vi "Clean Shutdown Check (SubVI).vi"(7 "System Message Queue In":refnum<queue>, 8 "error in (no error)":errorcluster) -> (0 "error out":errorcluster)   [LabVIEW 2019]
uses:
  Globals and Definitions/System Message.ctl
  Globals and Definitions/Initialization Globals.vi
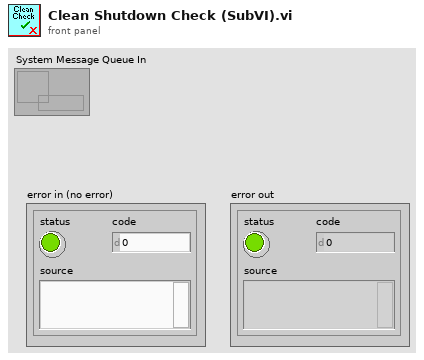
[diagram p1: front panel]
types:
  T1 = typedef "System Message.ctl" = cluster{"Message Tag":string, "Message Body":string, "Snooze Time (s)":dbl, "Snooze Alert?":bool, "Log Event?":bool, "Send Email":i32}
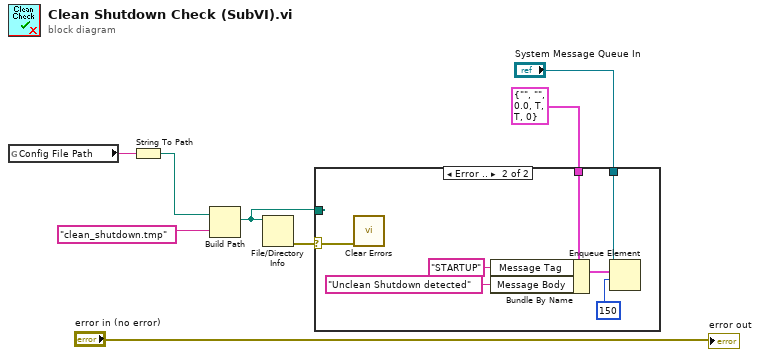
[diagram p0: block diagram]
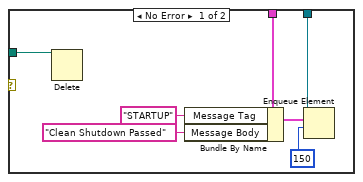
[diagram p2: hidden frame]
diagram:
  n1 = global read "Initialization Globals.vi" "Config File Path"() -> (w8:string)
  n2 = String To Path(string=w8) -> (path=w7:path)
  n3 = Build Path(base path=w7, name or relative path="clean_shutdown.tmp") -> (appended path=w3:path)
  n4 = File/Directory Info(path=w3) -> (error out=w2:errorcluster)  [unwired: 1 in, 6 out]
  n5 = case shown="Error .." w2 {
    selector: w2 -> [_ w22]
    tunnel: w3 -> [w15 _]
    tunnel: T1 {"Message Tag"="", "Message Body"="", "Snooze Time (s)"=0.0, "Snooze Alert?"=TRUE, "Log Event?"=TRUE, "Send Email"=0} -> [w10 w19]
    tunnel: "System Message Queue In" -> [w9 w18]
    frame No Error {
      n6 = Delete(path (use dialog)=w15) -> ()  [unwired: 4 in, 3 out]
      n7 = Bundle By Name(cluster=w10, "Message Tag"="STARTUP", "Message Body"="Clean Shutdown Passed") -> (w13:T1)
      n8 = Enqueue Element(queue=w9, element=w13, timeout in ms (-1)=150) -> ()  [unwired: 1 in, 3 out]
    }
    frame Error {
      n9 = call <vilib>:"Clear Errors.vi"("error in (no error)"=w22) -> ()  [unwired: 5 in, 2 out]
      n10 = Bundle By Name(cluster=w19, "Message Tag"="STARTUP", "Message Body"="Unclean Shutdown detected") -> (w20:T1)
      n11 = Enqueue Element(queue=w18, element=w20, timeout in ms (-1)=150) -> ()  [unwired: 1 in, 3 out]
    }
  }
  "error out" <- "error in (no error)"
